vi "ke37xx Is Closed.vi"(0 "VISA Resource Name":refnum<visa-resource-name>, 1 "Channel List":string, 11 "error in (no error)":errorcluster, 12 "Bytes To Read (1024)":u32=1024) -> (4 "VISA Resource Name Out":refnum<visa-resource-name>, 8 "Is Closed":bool[](array[boolean]), 15 "error out":errorcluster)   [LabVIEW 2009, in "Keithley 3700 Series.lvlib"]
doc: "This VI allows determine if a set of channels is closed or open."
uses:
  <instrlib>/Keithley 3706/Keithley 3700 Series.lvlib
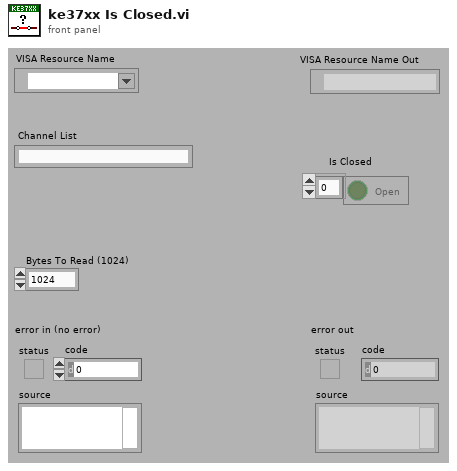
[diagram p1: front panel]
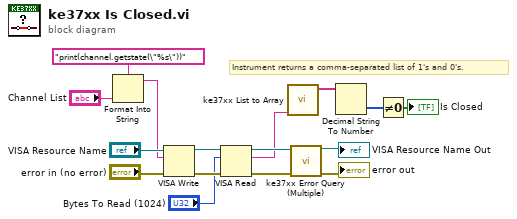
[diagram p0: block diagram]
diagram:
  # "Instrument returns a comma-separated list of 1's and 0's."
  n1 = Format Into String(format string="print(channel.getstate(\"%s\"))", "Channel List") -> (resulting string=w5:string)  [unwired: 2 in, 1 out]
  n2 = VISA Write(VISA resource name="VISA Resource Name", write buffer=w5, error in (no error)="error in (no error)") -> (VISA resource name out=w9:refnum<visa-resource-name>, error out=w8:errorcluster)  [unwired: 1 out]
  n3 = VISA Read(VISA resource name=w9, byte count="Bytes To Read (1024)", error in (no error)=w8) -> (VISA resource name out=w12:refnum<visa-resource-name>, read buffer=w1:string, error out=w11:errorcluster)  [unwired: 1 out]
  n4 = call <instrlib>:"ke37xx List to Array.vi"("List"=w1) -> ("Output String Array"=w4:string[])  [unwired: 1 in, 5 out]
  n5 = call <instrlib>:"ke37xx Error Query (Multiple).vi"("VISA resource name"=w12, "error in (no error)"=w11) -> ("VISA resource name out"=→"VISA Resource Name Out":refnum<visa-resource-name>, "error out"=→"error out":errorcluster)  [unwired: 12 out]
  n6 = Decimal String To Number(string=w4) -> (number=w3:i32[])  [unwired: 3 out]
  n7 = Not Equal To 0?(x=w3) -> (x != 0?=→"Is Closed":bool[])
